vi "Write SerialData.vi"(8 "error in (no error)":errorcluster, 10 "SerialData":refnum<class "Data.lvclass">[](array[class]), 11 "CRDS Data in":refnum<class "CRDS Data.lvclass">) -> (0 "error out":errorcluster, 3 "CRDS Data out":refnum<class "CRDS Data.lvclass">)   [LabVIEW 2014, in "CRDS Data.lvclass"]
uses:
  CRDS Data.lvclass
  Data/Data.lvclass
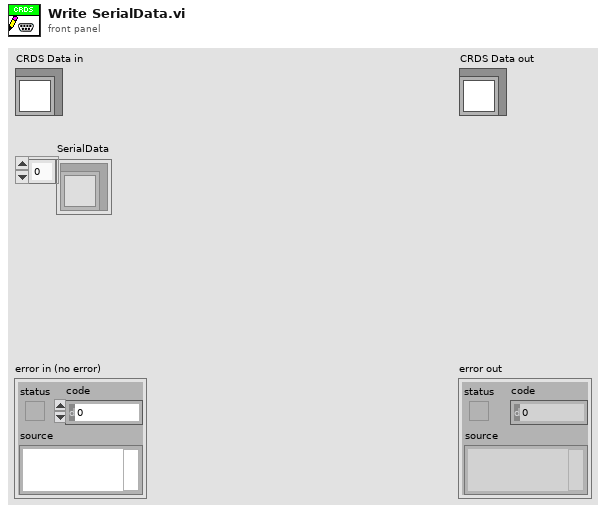
[diagram p1: front panel]
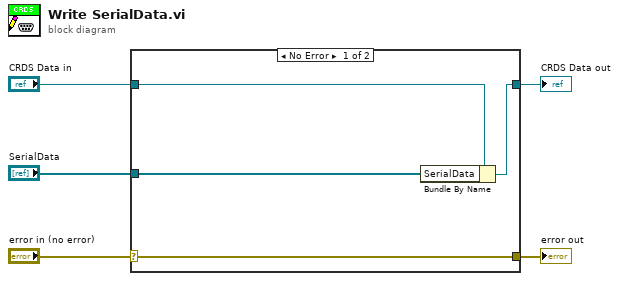
[diagram p0: block diagram]
diagram:
  n1 = case shown="No Error" "error in (no error)" {
    selector: "error in (no error)" -> [w9 w10]
    tunnel: [w9 w10] -> w4
    tunnel: [w7 w11] -> w2
    tunnel: "CRDS Data in" -> [w8 w11]
    tunnel: "SerialData" -> [w6 _]
    frame No Error {
      n2 = Bundle By Name(cluster=w8, "SerialData"=w6) -> (w7:refnum<class "CRDS Data.lvclass">)
    }
    frame Error {
    }
  }
  "error out" <- w4
  "CRDS Data out" <- w2
